vi "AutoRotatePID.vi"(9 "DesiredAngle":dbl format="%#_13g", 10 "ActualAngle":dbl format="%#_13g") -> (1 "TankDriveRight":dbl format="%.2f", 2 "TankDriveLeft":dbl format="%.2f")   [LabVIEW 2013]
doc: "Uses a PID to rotate the robot from the actual angle to the desired angle. The VI returns values for tank drive left and right which can be fed directly into tank drive."
uses:
  <vilib>/addons/control/pid/pid.llb/PID (DBL).vi
  <vilib>/addons/control/pid/NI_PID_pid.lvlib
panel:
  in  "reinitialize? (F)":bool
  in  "PID gains":T1={"proportional gain (Kc)"=1.0, "integral time (Ti, min)"=0.0, "derivative time (Td, min)"=0.0} {"derivative time (Td, min)" format="%.3f"; "integral time (Ti, min)" format="%.3f"; "proportional gain (Kc)" format="%.3f"}
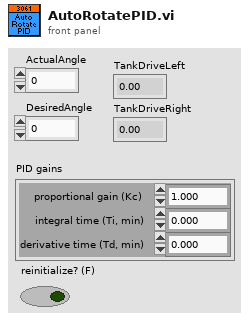
[diagram p1: front panel]
types:
  T1 = cluster{"proportional gain (Kc)":dbl, "integral time (Ti, min)":dbl, "derivative time (Td, min)":dbl}
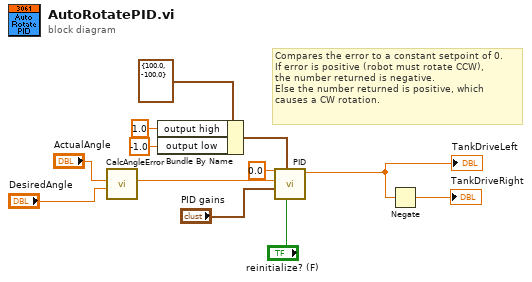
[diagram p0: block diagram]
diagram:
  # "Compares the error to a constant setpoint of 0.\nIf error is positive (robot must rotate CCW),\nthe number returned is negative.\nElse the number returned is positive, which\ncauses a CW rotation."
  n1 = call "CalcAngleError.vi"("DesiredAngle"="DesiredAngle", "ActualAngle"="ActualAngle") -> ("Error"=w1:dbl)  [unwired: 9 in]
  n2 = Bundle By Name(cluster=cluster{"output high":dbl, "output low":dbl} {"output high"=100.0, "output low"=-100.0} ("output range"), "output high"=1.0, "output low"=-1.0) -> (w9:cluster{"output high":dbl, "output low":dbl})
  n3 = call-poly <vilib>:"PID.vi"("reinitialize? (F)"="reinitialize? (F)", "output range"=w9, "PID gains"="PID gains", "process variable"=w1, "setpoint"=0.0) -> ("output"=w6:dbl)  [unwired: 5 in, 1 out]
  "TankDriveLeft" <- w6
  n4 = Negate(x=w6) -> (-x=→"TankDriveRight":dbl)
